vi "Write Scripts.vi"(8 "error in (no error)":errorcluster, 10 "Scripts":string, 11 "scripts manager in":refnum<class "scripts manager.lvclass">) -> (0 "error out":errorcluster, 3 "scripts manager out":refnum<class "scripts manager.lvclass">)   [LabVIEW 2016, in "scripts manager.lvclass"]
uses:
  scripts manager.lvclass
  scripts manager.lvclass/scripts manager.ctl
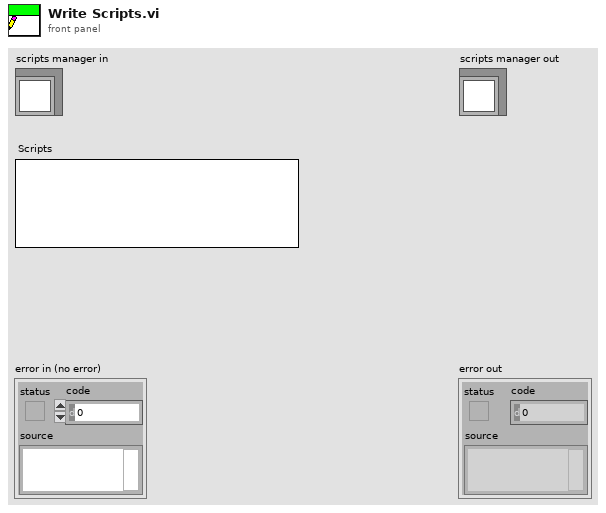
[diagram p1: front panel]
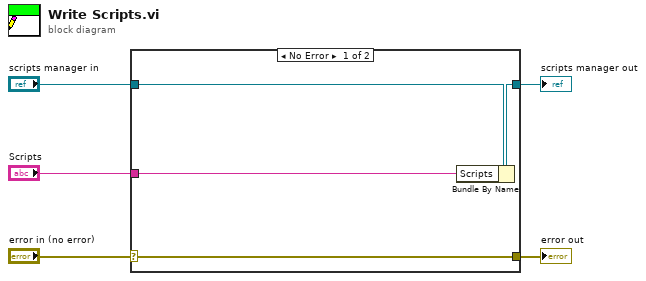
[diagram p0: block diagram]
diagram:
  n1 = case shown="No Error" "error in (no error)" {
    selector: "error in (no error)" -> [w9 w10]
    tunnel: [w9 w10] -> w4
    tunnel: [w7 w11] -> w2
    tunnel: "scripts manager in" -> [w8 w11]
    tunnel: "Scripts" -> [w6 _]
    frame No Error {
      n2 = Bundle By Name(cluster=w8, "Scripts"=w6) -> (w7:refnum<class "scripts manager.lvclass">)
    }
    frame Error {
    }
  }
  "error out" <- w4
  "scripts manager out" <- w2
